vi "HCC Folder Path.vi"() -> (3 "appended path":path)   [LabVIEW 2018]
uses:
  Utility/Save File/Save File.lvlib
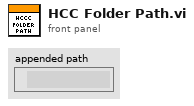
[diagram p1: front panel]
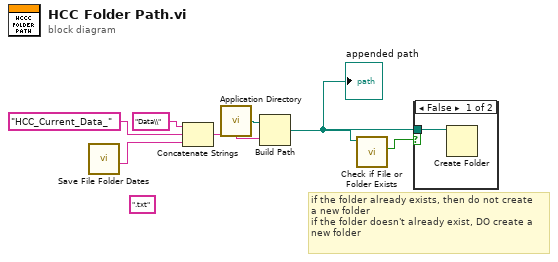
[diagram p0: block diagram]
diagram:
  (unwired) ".txt" ("string")
  # "if the folder already exists, then do not create\na new folder\nif the folder doesn't already exist, DO create a\nnew folder"
  n1 = call "Save File Folder Dates.vi"() -> ("Year/Month/Day"=w6:string)  [unwired: 8 in, 3 out]
  n2 = Concatenate Strings("Data\\" ("name or relative path"), "HCC_Current_Data_" ("string"), w6) -> (w7:string)
  n3 = call <vilib>:"Application Directory.vi"() -> ("Application Directory"=w3:path)
  n4 = Build Path(base path=w3, name or relative path=w7) -> (appended path=w2:path)
  "appended path" <- w2
  n5 = call <vilib>:"Check if File or Folder Exists.vi"("path"=w2) -> ("file or folder exists?"=w1:bool)  [unwired: 8 in, 2 out]
  n6 = case shown="False" w1 {
    tunnel: w2 -> [w8 _]
    frame False {
      n7 = Create Folder(path (use dialog)=w8) -> ()  [unwired: 2 in, 3 out]
    }
    frame True {
    }
  }
